vi "mode_comparison.vi"() -> ()   [LabVIEW 2015]
uses:
  <vilib>/Analysis/_algsub.llb/Matrix Norm Type.ctl
  <vilib>/Analysis/_algsub.llb/Real Matrix Norm.vi
  <vilib>/Analysis/NI_AALPro.lvlib
panel:
  out "Trace distance":dbl
  in  "stop":bool
  out "Difference":dbl[][](graph)
  in  "represented width & height (in m)":dbl=0.006 format="%#_6p"
  in  "x_centre (in m; default 0)":dbl step=0.0001 format="%.5f"
  in  "wavelength (in m)":dbl=7.1e-07 format="%#_6p"
  in  "beam waist w0 (in m; default 1E-4 = 0.1mm)":dbl=0.0005 format="%.2p"
  in  "y_centre (in m; default 0)":dbl step=0.0001 format="%.5f"
  in  "modes":T1(array[cluster])=[{"type"=enum."LG mode", "m or L"=-2, "n or p"=0, "weight"=0.7071, "phase"=0.0}, {"type"=enum."LG mode", "m or L"=2, "n or p"=0, "weight"=0.7071, "phase"=0.0}]
  out "Image":dbl[][](graph)
  in  "input image":path
  out "Simulation":dbl[][](graph)
  out "mode superposition":T2={"amplitude matrix"=array600x600[360000 elements], "number of columns in amplitude matrix"=600, "number of rows in amplitude matrix"=600, "represented width (in m)"=0.006, "represented height (in m)"=0.006, "wavelength (in m)"=7.1e-07}
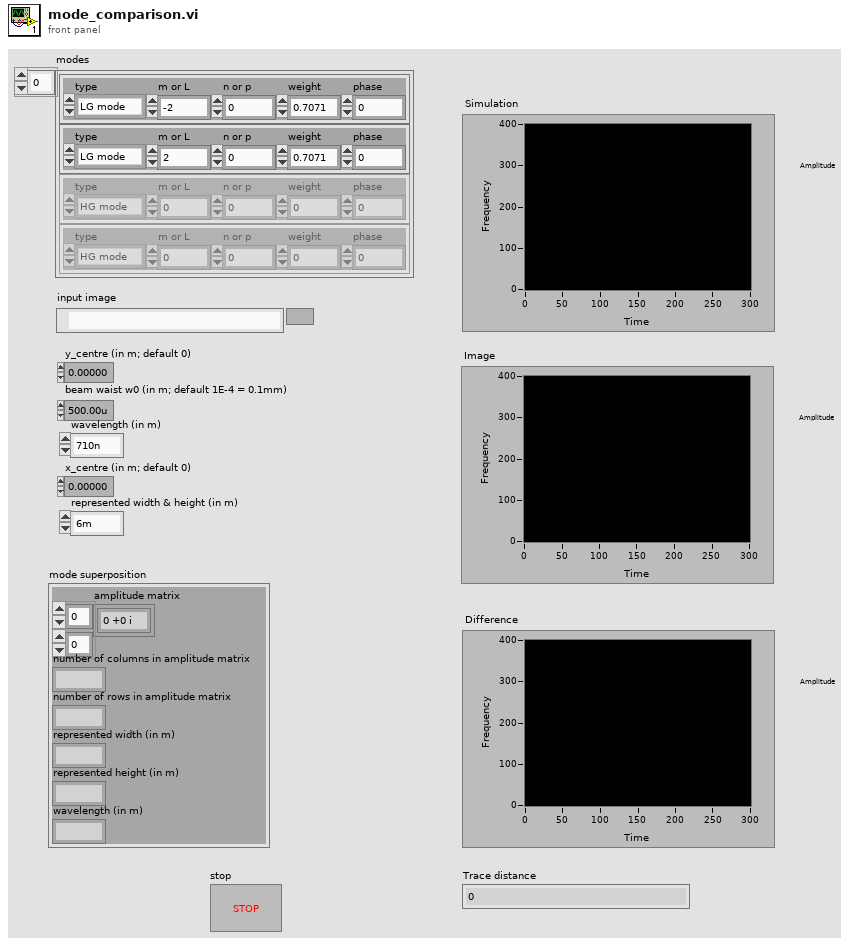
[diagram p1: front panel]
types:
  T1 = cluster{"type":enum16{"HG mode", "LG mode"}, "m or L":i32, "n or p":i32, "weight":dbl, "phase":dbl}[]
  T2 = cluster{"amplitude matrix":cdb[][], "number of columns in amplitude matrix":i32, "number of rows in amplitude matrix":i32, "represented width (in m)":dbl, "represented height (in m)":dbl, "wavelength (in m)":dbl}
  T3 = typedef "NI_AALPro.lvlib/Matrix Norm Type.ctl" = i32
  T4 = typedef "imagedata.ctl" = cluster{"image type":i32, "image depth":i32, "image":u8[], "mask":u8[], "colors":u32[], "Rectangle":cluster{"left":i16, "top":i16, "right":i16, "bottom":i16}}
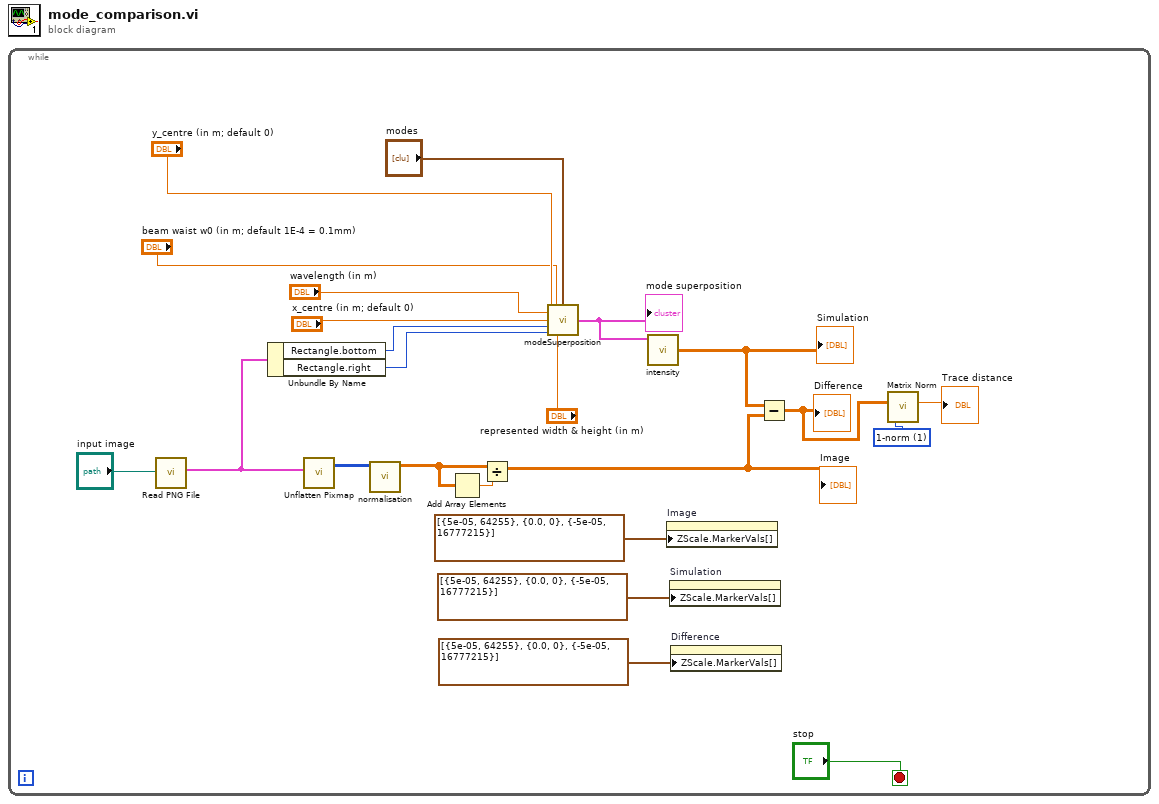
[diagram p0: block diagram]
diagram:
  n1 = while {
    stop <- "stop" stop-if-true
    w3 = T3 1 items=["2-norm", "1-norm", "F-norm", "Inf-norm"] ("norm type")
    n2 = call <vilib>:"Read PNG File.vi"("path to PNG file"="input image") -> ("image data"=w18:T4)  [unwired: 8 in, 2 out]
    n3 = Unbundle By Name(w18) -> ("Rectangle.bottom"=w16:i16, "Rectangle.right"=w15:i16)
    n4 = call <vilib>:"Unflatten Pixmap.vi"("image data"=w18) -> ("24-bit pixmap"=w21:u32[][])  [unwired: 4 in, 6 out]
    n5 = call "normalisation.vi"("intensity matrix"=w21) -> ("Array"=w20:dbl[][])  [unwired: 10 in]
    n6 = Add Array Elements(numeric array=w20) -> (sum=w19:dbl)
    n7 = Divide(x=w20, y=w19) -> (x/y=w9:dbl[][])
    "Image" <- w9
    n8 = call <userlib>:"modeSuperposition.vi"("y_centre (in m; default 0)"="y_centre (in m; default 0)", "modes"="modes", "beam waist w0 (in m; default 1E-4 = 0.1mm)"="beam waist w0 (in m; default 1E-4 = 0.1mm)", "number of columns in amplitude matrix"=w16, "wavelength (in m)"="wavelength (in m)", "number of rows in amplitude matrix"=w15, "x_centre (in m; default 0)"="x_centre (in m; default 0)", "represented width & height (in m)"="represented width & height (in m)") -> ("mode superposition"=w23:T2)
    "mode superposition" <- w23
    n9 = call <userlib>:"intensity.vi"("beam cluster"=w23) -> ("intensity matrix"=w2:dbl[][])
    "Simulation" <- w2
    n10 = property on="Image" class="IntGraph (strict)"("ZScale.MarkerVals[]"=cluster{dbl, u32}[] [{5e-05, 64255}, {0.0, 0}, {-5e-05, 16777215}] ("Z Scale.Marker Values[]")) -> ()  [unwired: 2 in, 2 out]
    n11 = property on="Simulation" class="IntGraph (strict)"("ZScale.MarkerVals[]"=cluster{dbl, u32}[] [{5e-05, 64255}, {0.0, 0}, {-5e-05, 16777215}] ("Z Scale.Marker Values[]")) -> ()  [unwired: 2 in, 2 out]
    n12 = property on="Difference" class="IntGraph (strict)"("ZScale.MarkerVals[]"=cluster{dbl, u32}[] [{5e-05, 64255}, {0.0, 0}, {-5e-05, 16777215}] ("Z Scale.Marker Values[]")) -> ()  [unwired: 2 in, 2 out]
    n13 = Subtract(x=w2, y=w9) -> (x-y=w4:dbl[][])
    "Difference" <- w4
    n14 = call-poly <vilib>:"Matrix Norm.vi"("norm type"=w3, "Input Matrix"=w4) -> ("norm"=→"Trace distance":dbl)  [unwired: 1 out]
  }
